vi "New Custom Sink.vi"(8 "error in (no error)":errorcluster, 11 "Button Name":string) -> (0 "error out":errorcluster, 3 "Custom Sink out":refnum<class "Custom Sink.lvclass">)   [LabVIEW 2020, in "Custom Sink.lvclass"]
uses:
  Custom Sink.lvclass
  Custom Sink.lvclass/Custom Sink.ctl
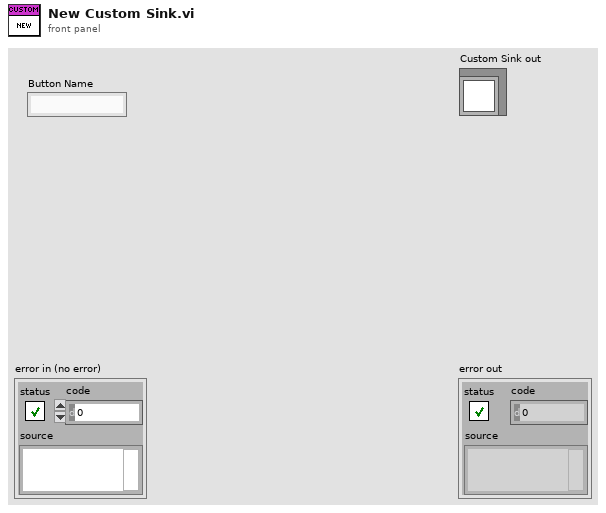
[diagram p1: front panel]
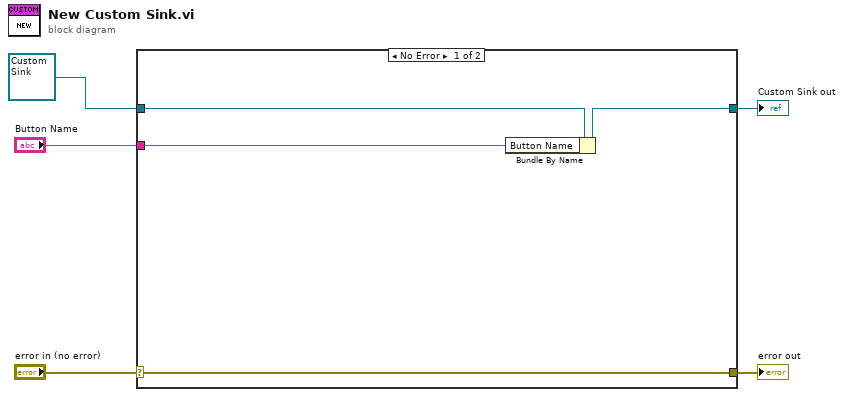
[diagram p0: block diagram]
diagram:
  n1 = case shown="No Error" "error in (no error)" {
    selector: "error in (no error)" -> [w9 w11]
    tunnel: [w9 w11] -> w4
    tunnel: [w7 w10] -> w2
    tunnel: refnum<class "Custom Sink.lvclass"> refnum ("Custom Sink in") -> [w8 w10]
    tunnel: "Button Name" -> [w6 _]
    frame No Error {
      n2 = Bundle By Name(cluster=w8, "Button Name"=w6) -> (w7:refnum<class "Custom Sink.lvclass">)
    }
    frame Error {
    }
  }
  "error out" <- w4
  "Custom Sink out" <- w2
